vi "7HP_EnFlo_Specific - USB.vi"(5 "Datalog file path (full)":path, 6 "COM port":refnum<visa-resource-name>, 7 "Log data stream":bool, 8 "Set data rate (Hz)":u8(ring)=14 items=["1", "2", "4", "5", "8", "10", "16", "20", "25", "32", "40", "50", "64", "80", "100", "125", "160", "200", "250", "320", "400", "500", "625", "800", "1000"], 9 "N samples":u32=1000, 10 "Command":T2="s") -> (0 "Error":errorcluster, 2 "All samples out":sgl[][](array[numeric]), 3 "Rendezvous out":bool)   [LabVIEW 2020]
uses:
  ctls/7HP_Cmd (USB).ctl
  Globals/Meas_global.vi
panel:
  in  "Main":T1(tab)
  out "Serial number":u32 format="%0d"
  out "Pressure sensor EEPROM checksums ok":bool[](array[boolean])
  out "Pressure sensor temperatures in range":bool[](array[boolean])
  out "Pressure sensor values in range":bool[](array[boolean])
  out "Subsystems ok":bool[](array[boolean])
  out "n":u16
  out "Auto zero progBar":u16(slide) caption="Collecting samples, please maintain dP = 0" scale=0.0..1000.0
  out "P_raw_Azero":sgl[](array[numeric])
  in  "EEPROM array 2":u16[](array[numeric])
  in  "EEPROM array":sgl[](array[numeric])
  out "Chk ok":bool
  out "EEPROM Checksum":u16 format="%04x"
  out "received":bool
  out "Returned data rate (Hz)":u16
  out "sent":bool
  out "Pitch (deg)":sgl format="%.2f"
  out "Roll (deg)":sgl format="%.2f"
  out "frm err":u32
  out "chk err":u32
  in  "Stop Data":bool
  out "Relative humidity (%)":sgl
  out "Env. sensor die temperature (deg C)":sgl
  out "External thermistor temperature (deg C)":sgl
  out "Atmospheric pressure (mbar)":sgl
  out "Checksum ok":bool
  out "Gyration vector (deg / s)":sgl[](array[numeric])
  out "Acceleration vector (g)":sgl[](array[numeric])
  out "Pressures":sgl[][](graph)
  out "Stream enabled":bool
  # "Paul Nathan 10/2020"
  # "Output array order:\nP0.... (Pa)\n.\n.\nP6.... (Pa)\nP_atmos (mbar)....\nT_ext (deg C)....\nT_env (deg C)....\nRH (%)....\nax (g)....\nay (g)....\naz (g)....\nwx (deg / s)....\nwy (deg / s)....\nwz (deg / s)...."
  # "Pressure sensor 0 EEPROM checksum okay"
  # "Pressure sensor 1 EEPROM checksum okay"
  # "Pressure sensor 2 EEPROM checksum okay"
  # "Pressure sensor 3 EEPROM checksum okay"
  # "Pressure sensor 4 EEPROM checksum okay"
  # "Pressure sensor 5 EEPROM checksum okay"
  # "Pressure sensor 6 EEPROM checksum okay"
  # "Pressure sensor 0 temperature in range"
  # "Pressure sensor 1 temperature in range"
  # "Pressure sensor 2 temperature in range"
  # "Pressure sensor 3 temperature in range"
  # "Pressure sensor 4 temperature in range"
  # "Pressure sensor 5 temperature in range"
  # "Pressure sensor 6 temperature in range"
  # "Pressure sensor 0 value in range"
  # "Pressure sensor 1 value in range"
  # "Pressure sensor 2 value in range"
  # "Pressure sensor 3 value in range"
  # "Pressure sensor 4 value in range"
  # "Pressure sensor 5 value in range"
  # "Pressure sensor 6 value in range"
  # "Environmental sensor present"
  # "Inertial sensor present"
  # "Accelerometer self test pass"
  # "Gyroscope self test pass"
  # "External thermistor value in range"
  # "MCU EEPROM checksum ok"
  # "of 1000"
  # "P0 raw auto-zero"
  # "P1 raw auto-zero"
  # "P2 raw auto-zero"
  # "P3 raw auto-zero"
  # "P4 raw auto-zero"
  # "P5 raw auto-zero"
  # "P6 raw auto-zero"
  # "Power-up defaults"
  # "P0 raw auto-zero"
  # "Data rate (Hz)"
  # "P1 raw auto-zero"
  # "TTL streaming"
  # "P2 raw auto-zero"
  # "USB streaming"
  # "P3 raw auto-zero"
  # "TTL stream contains full data"
  # "P4 raw auto-zero"
  # "Accelerometer range mode"
  # "P5 raw auto-zero"
  # "Gyroscope range mode"
  # "P6 raw auto-zero"
  # "IMU rate mode"
  # "Atmospheric pressure offset (Pa)"
  # "External thermistor temperature offset (deg C)"
  # "Serial number"
  # "TTL baud rate (bps)"
  # "Accelerometer vector magnitude scale factor"
  # "Gyroscope x component offset (deg / s)"
  # "Gyroscope y component offset (deg / s)"
  # "Gyroscope z component offset (deg / s)"
  # "w_x"
  # "w_y"
  # "w_z"
  # "a_x"
  # "a_y"
  # "a_z"
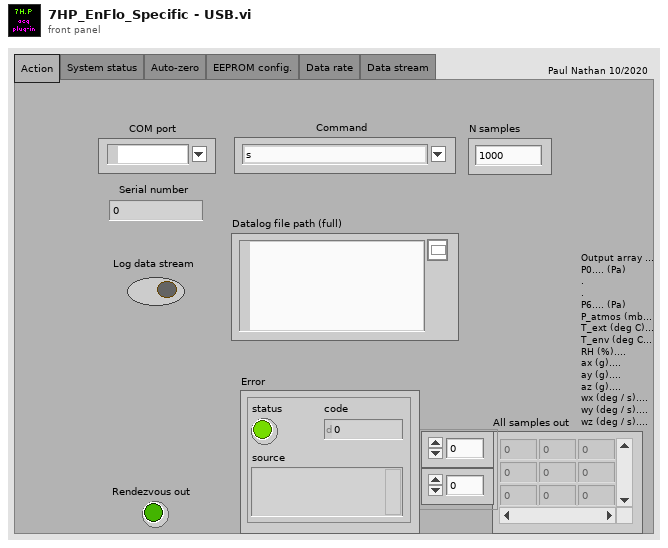
[diagram p1: front panel]
types:
  T1 = enum32{"Action", "System status", "Auto-zero", "EEPROM config.", "Data rate", "Data stream"}
  T2 = typedef "7HP_Cmd (USB).ctl" = string
  T3 = enum16{"open", "replace", "create", "open or create", "replace or create", "replace or create with confirmation"}
  T4 = typedef "Rendezvous RefNum" = refnum<k1>
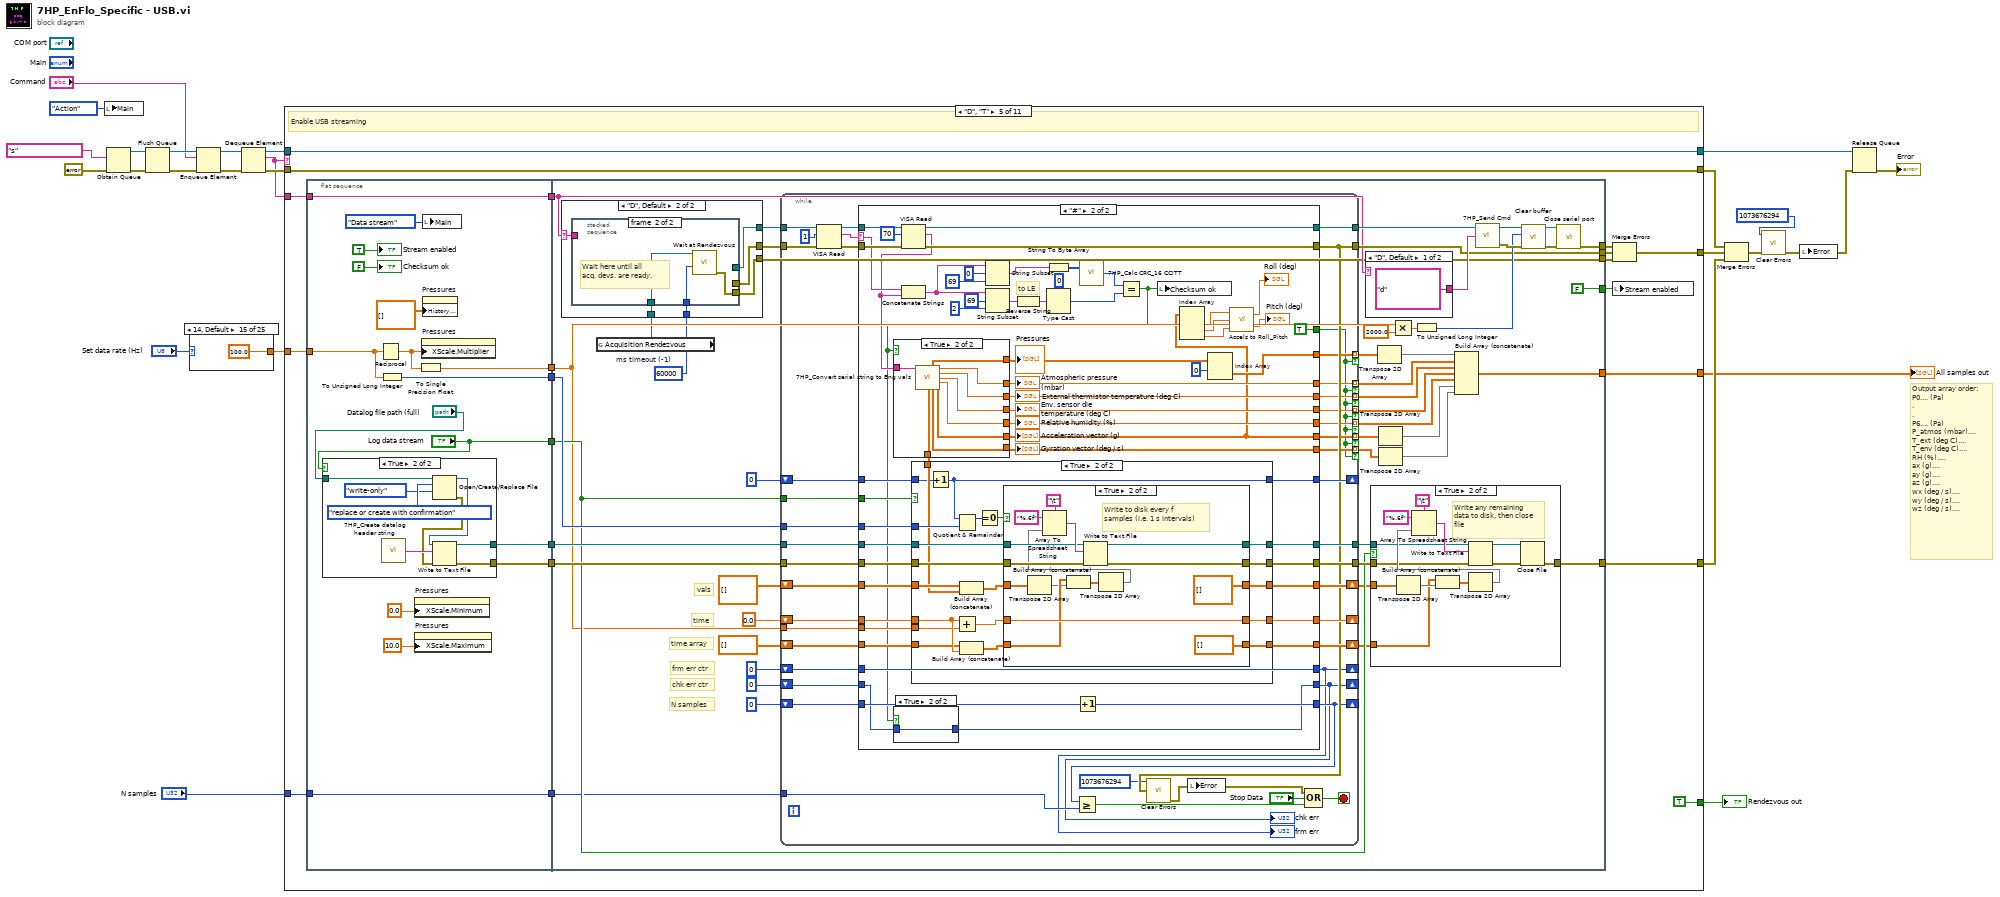
[diagram p0: block diagram]
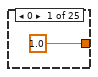
[diagram p2: hidden frame]
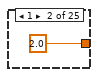
[diagram p3: hidden frame]
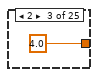
[diagram p4: hidden frame]
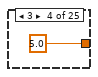
[diagram p5: hidden frame]
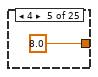
[diagram p6: hidden frame]
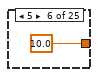
[diagram p7: hidden frame]
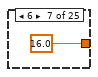
[diagram p8: hidden frame]
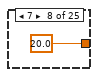
[diagram p9: hidden frame]
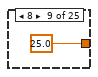
[diagram p10: hidden frame]
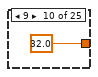
[diagram p11: hidden frame]
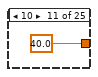
[diagram p12: hidden frame]
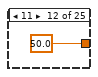
[diagram p13: hidden frame]
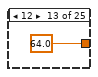
[diagram p14: hidden frame]
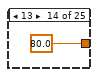
[diagram p15: hidden frame]
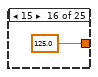
[diagram p16: hidden frame]
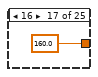
[diagram p17: hidden frame]
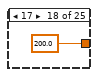
[diagram p18: hidden frame]
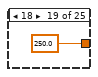
[diagram p19: hidden frame]
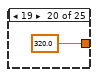
[diagram p20: hidden frame]
diagram:
  # "Output array order:\nP0.... (Pa)\n.\n.\nP6.... (Pa)\nP_atmos (mbar)....\nT_ext (deg C)....\nT_env (deg C)....\nRH (%)....\nax (g)....\nay (g)....\naz (g)....\nwx (deg / s)....\nwy (deg / s)....\nwz (deg / s)...."
  n1 = local write "Main"(T1."Action" ("Main")) -> ()
  n2 = Obtain Queue(element data type=T2 "s" ("Combo Box"), error in (no error)=errorcluster {"status"=FALSE, "code"=0, "source"=""}) -> (queue out=w24:refnum<queue>, error out=w25:errorcluster)  [unwired: 3 in, 1 out]
  n3 = Flush Queue(queue=w24, error in (no error)=w25) -> (queue out=w23:refnum<queue>, error out=w18:errorcluster)  [unwired: 1 out]
  n4 = case shown="14, Default" "Set data rate (Hz)" {
    tunnel: [1.0 2.0 4.0 5.0 8.0 10.0 16.0 20.0 25.0 32.0 40.0 50.0 64.0 80.0 100.0 125.0 160.0 200.0 250.0 320.0 400.0 500.0 625.0 800.0 1000.0] -> w3
    frame 0 {
    }
    frame 1 {
    }
    frame 2 {
    }
    frame 3 {
    }
    frame 4 {
    }
    frame 5 {
    }
    frame 6 {
    }
    frame 7 {
    }
    frame 8 {
    }
    frame 9 {
    }
    frame 10 {
    }
    frame 11 {
    }
    frame 12 {
    }
    frame 13 {
    }
    frame 14, Default {
    }
    frame 15 {
    }
    frame 16 {
    }
    frame 17 {
    }
    frame 18 {
    }
    frame 19 {
    }
    frame 20 {
    }
    frame 21 {
    }
    frame 22 {
    }
    frame 23 {
    }
    frame 24 {
    }
  }
  n5 = Enqueue Element(queue=w23, element="Command", error in (no error)=w18) -> (queue out=w19:refnum<queue>, error out=w17:errorcluster)  [unwired: 1 in, 1 out]
  n6 = Dequeue Element(queue=w19, error in (no error)=w17) -> (queue out=w14:refnum<queue>, element=w12:T2, error out=w13:errorcluster)  [unwired: 1 in, 1 out]
  n7 = case shown="\"D\", \"T\"" w12 {
    tunnel: w14 -> [w57 w96 w133 w210 w285 w592 w616 w670 w703 w726 w730]
    tunnel: [w57 w96 w133 w210 w285 w592 w616 w670 w703 w726 w730] -> w15
    tunnel: w13 -> [w56 w95 w132 w209 w284 w591 w617 w671 w702 w725 w729]
    tunnel: [w56 w95 w132 w209 w284 w591 w617 w671 w702 w725 w729] -> w11
    tunnel: w12 -> [w55 w94 w131 w208 w283 w594 w619 w673 w701 _ _]
    tunnel: [w53 w92 w129 w206 w268 w593 w618 w672 w699 errorcluster {"status"=FALSE, "code"=0, "source"=""} ("Error out") errorcluster {"status"=FALSE, "code"=0, "source"=""} ("Error out")] -> w10
    tunnel: [_ _ _ _ w281 _ _ _ _ _ _] -> w9
    tunnel: "N samples" -> [_ _ _ _ w274 _ _ _ _ _ _]
    tunnel: [_ _ _ _ w272 _ _ _ _ _ _] -> w5
    tunnel: w3 -> [_ _ _ _ w271 w589 _ _ _ _ _]
    tunnel: [FALSE FALSE FALSE FALSE TRUE FALSE FALSE FALSE FALSE FALSE FALSE] -> w1
    frame "S", "s" {
      # "Perform self-test and retrieve status bytes, Retrieve status bytes"
      n8 = flat-sequence {
        tunnel: w55 -> [w60]
        tunnel: [w60] -> w54
        tunnel: w54 -> [w66]
        tunnel: [w61] -> w53
        frame #0 {
          w59 = bool[] [] ("Pressure sensor EEPROM checksums ok")
          n9 = local write "Main"(T1."System status" ("Main")) -> ()
          "Pressure sensor EEPROM checksums ok" <- w59
          "Pressure sensor temperatures in range" <- w59
          "Pressure sensor values in range" <- w59
          "Subsystems ok" <- w59
        }
        frame #1 {
          w70 = 1 ("length (rest)")
          w78 = u8 0 ("byte count")
          n10 = local read "COM port"() -> (w67:refnum<visa-resource-name>)
          n11 = call "Open serial port.vi"("timeout (ms)"=u32 5000, "VISA resource name"=w67) -> ("Error out"=w88:errorcluster, "VISA resource name out"=w89:refnum<visa-resource-name>)  [unwired: 8 in]
          n12 = call "7HP_Send Cmd.vi"("Error In"=w88, "Operation"=w66, "Port"=w89) -> ("Error Out"=w86:errorcluster, "Port out"=w87:refnum<visa-resource-name>)  [unwired: 1 in]
          n13 = VISA Read(VISA resource name=w87, byte count=u32 4, error in (no error)=w86) -> (VISA resource name out=w84:refnum<visa-resource-name>, read buffer=w73:string, error out=w83:errorcluster)  [unwired: 1 out]
          n14 = call "Close serial port.vi"("Error in"=w83, "VISA resource name"=w84) -> ("Error out"=w61:errorcluster)  [unwired: 9 in]
          n15 = String Subset(string=w73, offset (0)=0, length (rest)=w70) -> (substring=w82:string)
          n16 = String Subset(string=w73, offset (0)=1, length (rest)=w70) -> (substring=w81:string)
          n17 = String Subset(string=w73, offset (0)=2 ("length (rest)"), length (rest)=w70) -> (substring=w80:string)
          n18 = String Subset(string=w73, offset (0)=3, length (rest)=w70) -> (substring=w79:string)
          n19 = Type Cast(type=w78, x=w82) -> (*(type *) &x=w77:u8)
          n20 = Type Cast(type=w78, x=w81) -> (*(type *) &x=w76:u8)
          n21 = Type Cast(type=w78, x=w80) -> (*(type *) &x=w75:u8)
          n22 = Type Cast(type=w78, x=w79) -> (*(type *) &x=w74:u8)
          n23 = Number To Boolean Array(number=w77) -> (Boolean array=w65:bool[])
          n24 = Number To Boolean Array(number=w76) -> (Boolean array=w64:bool[])
          n25 = Number To Boolean Array(number=w75) -> (Boolean array=w63:bool[])
          n26 = Number To Boolean Array(number=w74) -> (Boolean array=w62:bool[])
          n27 = local write "Pressure sensor EEPROM checksums ok"(w65) -> ()
          n28 = local write "Pressure sensor temperatures in range"(w64) -> ()
          n29 = local write "Pressure sensor values in range"(w63) -> ()
          n30 = local write "Subsystems ok"(w62) -> ()
        }
      }
    }
    frame "Z", "z" {
      # "Perform permanent auto-zero (write values to EEPROM), Perform temporary auto-zero"
      n31 = flat-sequence {
        tunnel: w94 -> [w100]
        tunnel: [w100] -> w93
        tunnel: w93 -> [w107]
        tunnel: [w103] -> w92
        frame #0 {
          n32 = local write "Main"(T1."Auto-zero" ("Main")) -> ()
          "P_raw_Azero" <- sgl[] [] ("P_raw_Azero")
          "Auto zero progBar" <- u16 0 ("Collecting samples, please maintain dP = 0")
        }
        frame #1 {
          n33 = local read "COM port"() -> (w108:refnum<visa-resource-name>)
          n34 = call "Open serial port.vi"("timeout (ms)"=u32 16000, "VISA resource name"=w108) -> ("Error out"=w114:errorcluster, "VISA resource name out"=w115:refnum<visa-resource-name>)  [unwired: 8 in]
          n35 = call "7HP_Send Cmd.vi"("Error In"=w114, "Operation"=w107, "Port"=w115) -> ("Error Out"=w112:errorcluster, "Port out"=w113:refnum<visa-resource-name>)  [unwired: 1 in]
          n36 = VISA Read(VISA resource name=w113, byte count=u32 28, error in (no error)=w112) -> (VISA resource name out=w110:refnum<visa-resource-name>, read buffer=w104:string, error out=w109:errorcluster)  [unwired: 1 out]
          n37 = for {
            N: 1000 -> [_]
            shift-right: [w117] -> _
            shift-left: u16 0 -> [w118]
            n38 = Increment(x=w118) -> (x+1=w117:u16)
            "n" <- w117
            n39 = Wait (ms)(milliseconds to wait=u32 11) -> ()  [unwired: 1 out]
            n40 = local write "Auto zero progBar"(w117) -> ()
          }
          n41 = for {
            N: 7 -> [_]
            tunnel: [w121] -> w106 mode=indexing
            tunnel: w104 -> [w120]
            i -> [w127]
            w125 = 4 ("x")
            # "to BE"
            n42 = Multiply(x=w125, y=w127) -> (x*y=w126:i32)
            n43 = String Subset(string=w120, offset (0)=w126, length (rest)=w125) -> (substring=w124:string)
            n44 = Reverse String(1:w124) -> (0:w123:string)
            n45 = Type Cast(type=sgl 0.0 ("byte count"), x=w123) -> (*(type *) &x=w121:sgl)
          }
          n46 = call "Close serial port.vi"("Error in"=w109, "VISA resource name"=w110) -> ("Error out"=w103:errorcluster)  [unwired: 9 in]
          n47 = local write "P_raw_Azero"(w106) -> ()
        }
      }
    }
    frame "R" {
      # "Read all EEPROM values"
      n48 = flat-sequence {
        tunnel: w131 -> [w137]
        tunnel: [w137] -> w130
        tunnel: w130 -> [w175]
        tunnel: [w174] -> w129
        frame #0 {
          n49 = local write "EEPROM array"(sgl[] [] ("EEPROM array")) -> ()
          n50 = local write "Main"(T1."EEPROM config." ("Main")) -> ()
          n51 = local write "EEPROM array 2"(u16[] [] ("EEPROM array 2")) -> ()
        }
        frame #1 {
          # "to BE"
          # "to BE"
          n52 = local read "COM port"() -> (w176:refnum<visa-resource-name>)
          n53 = call "Open serial port.vi"("timeout (ms)"=u32 5000, "VISA resource name"=w176) -> ("Error out"=w182:errorcluster, "VISA resource name out"=w183:refnum<visa-resource-name>)  [unwired: 8 in]
          n54 = call "7HP_Send Cmd.vi"("Error In"=w182, "Operation"=w175, "Port"=w183) -> ("Error Out"=w180:errorcluster, "Port out"=w181:refnum<visa-resource-name>)  [unwired: 1 in]
          n55 = VISA Read(VISA resource name=w181, byte count=u32 70, error in (no error)=w180) -> (VISA resource name out=w178:refnum<visa-resource-name>, read buffer=w142:string, error out=w177:errorcluster)  [unwired: 1 out]
          n56 = call "Close serial port.vi"("Error in"=w177, "VISA resource name"=w178) -> ("Error out"=w174:errorcluster)  [unwired: 9 in]
          n57 = String Subset(string=w142, offset (0)=0, length (rest)=48 ("length (rest)")) -> (substring=w145:string)
          n58 = String Subset(string=w142, offset (0)=56, length (rest)=12 ("length (rest)")) -> (substring=w150:string)
          n59 = String Subset(string=w142, offset (0)=48, length (rest)=2 ("length (rest)")) -> (substring=w159:string)
          n60 = String Subset(string=w142, offset (0)=50, length (rest)=6 ("length (rest)")) -> (substring=w163:string)
          n61 = String Subset(string=w142, offset (0)=68, length (rest)=2 ("length (rest)")) -> (substring=w170:string)
          n62 = String Subset(string=w142, offset (0)=0, length (rest)=68 ("length (rest)")) -> (substring=w173:string)
          n63 = for {
            N: 12 -> [_]
            tunnel: [w196] -> w151 mode=indexing
            tunnel: w145 -> [w195]
            i -> [w200]
            w198 = 4 ("x")
            # "to BE"
            n64 = Multiply(x=w198, y=w200) -> (x*y=w199:i32)
            n65 = String Subset(string=w195, offset (0)=w199, length (rest)=w198) -> (substring=w194:string)
            n66 = Reverse String(1:w194) -> (0:w193:string)
            n67 = Type Cast(type=sgl 0.0 ("byte count"), x=w193) -> (*(type *) &x=w196:sgl)
          }
          n68 = for {
            N: 3 -> [_]
            tunnel: [w188] -> w152 mode=indexing
            tunnel: w150 -> [w187]
            i -> [w192]
            w190 = 4 ("x")
            # "to BE"
            n69 = Multiply(x=w190, y=w192) -> (x*y=w191:i32)
            n70 = String Subset(string=w187, offset (0)=w191, length (rest)=w190) -> (substring=w186:string)
            n71 = Reverse String(1:w186) -> (0:w185:string)
            n72 = Type Cast(type=sgl 0.0 ("byte count"), x=w185) -> (*(type *) &x=w188:sgl)
          }
          n73 = Reverse String(1:w159) -> (0:w153:string)
          n74 = Reverse String(1:w170) -> (0:w166:string)
          n75 = String To Byte Array(string=w173) -> (unsigned byte array=w164:u8[])
          n76 = call "7HP_Calc CRC_16 CCITT.vi"("Data bytes"=w164) -> ("CRC_16-CCITT"=w165:u16)  [unwired: 1 in]
          n77 = Type Cast(type=u16 0 ("byte count"), x=w153) -> (*(type *) &x=w160:u16)
          n78 = Type Cast(type=u16 0 ("byte count"), x=w166) -> (*(type *) &x=w139:u16)
          n79 = String To Byte Array(string=w163) -> (unsigned byte array=w161:u8[])
          n80 = To Unsigned Word Integer(number=w161) -> (unsigned 16bit integer=w162:u16[])
          n81 = Equal?(x=w139, y=w165) -> (x = y?=w138:bool)
          n82 = Build Array (concatenate)(w151, w152) -> (w140:sgl[])
          n83 = Build Array (concatenate)(w160, w162) -> (w141:u16[])
          n84 = local write "EEPROM array"(w140) -> ()
          n85 = local write "EEPROM array 2"(w141) -> ()
          n86 = local write "EEPROM Checksum"(w139) -> ()
          n87 = local write "Chk ok"(w138) -> ()
        }
      }
    }
    frame "W" {
      # "Write all EEPROM values (including new checksum)"
      n88 = flat-sequence {
        tunnel: w208 -> [w223]
        tunnel: [w223] -> w207
        tunnel: [w216] -> w204
        tunnel: [w213] -> w203
        tunnel: [w212] -> w202
        tunnel: [w211] -> w201
        tunnel: w207 -> [w249]
        tunnel: [w248] -> w206
        tunnel: w204 -> [w229]
        tunnel: w203 -> [w226]
        tunnel: w202 -> [w228]
        tunnel: w201 -> [w227]
        frame #0 {
          n89 = local write "Main"(T1."EEPROM config." ("Main")) -> ()
          n90 = Split 1D Array(array="EEPROM array", index=12) -> (first subarray=w216:sgl[], second subarray=w213:sgl[])
          n91 = Split 1D Array(array="EEPROM array 2", index=1) -> (first subarray=w219:u16[], second subarray=w220:u16[])
          n92 = Index Array(array=w219, index=0) -> (element=w212:u16)
          n93 = To Unsigned Byte Integer(number=w220) -> (unsigned 8bit integer=w211:u8[])
        }
        frame #1 {
          # "to LE"
          # "to LE"
          n94 = local read "COM port"() -> (w250:refnum<visa-resource-name>)
          n95 = for {
            N: 12 -> [_]
            tunnel: w229 -> [w262] mode=indexing
            shift-right: [w263] -> w233
            shift-left: "" -> [w264]
            # "to LE"
            n96 = Type Cast(type="", x=w262) -> (*(type *) &x=w261:string)
            n97 = Reverse String(1:w261) -> (0:w260:string)
            n98 = Concatenate Strings(w264, w260) -> (w263:string)
          }
          n99 = for {
            N: 3 -> [_]
            tunnel: w226 -> [w256] mode=indexing
            shift-right: [w257] -> w240
            shift-left: "" -> [w258]
            # "to LE"
            n100 = Type Cast(type="", x=w256) -> (*(type *) &x=w255:string)
            n101 = Reverse String(1:w255) -> (0:w254:string)
            n102 = Concatenate Strings(w258, w254) -> (w257:string)
          }
          n103 = Type Cast(type="", x=w228) -> (*(type *) &x=w237:string)
          n104 = Reverse String(1:w237) -> (0:w239:string)
          n105 = call "Open serial port.vi"("timeout (ms)"=u32 5000, "VISA resource name"=w250) -> ("Error out"=w251:errorcluster, "VISA resource name out"=w252:refnum<visa-resource-name>)  [unwired: 8 in]
          n106 = Byte Array To String(unsigned byte array=w227) -> (string=w241:string)
          n107 = Concatenate Strings(w233, w239, w241, w240) -> (w234:string)
          n108 = String To Byte Array(string=w234) -> (unsigned byte array=w242:u8[])
          n109 = call "7HP_Calc CRC_16 CCITT.vi"("Data bytes"=w242) -> ("CRC_16-CCITT"=w224:u16)  [unwired: 1 in]
          "EEPROM Checksum" <- w224
          n110 = Type Cast(type="", x=w224) -> (*(type *) &x=w243:string)
          n111 = Reverse String(1:w243) -> (0:w244:string)
          n112 = Concatenate Strings(w234, w244) -> (w225:string)
          n113 = call "7HP_Send Cmd + Data.vi"("Error In"=w251, "Data"=w225, "Operation"=w249, "Port"=w252) -> ("Error Out"=w247:errorcluster, "Port out"=w246:refnum<visa-resource-name>)  [unwired: 1 in]
          n114 = call "Close serial port.vi"("Error in"=w247, "VISA resource name"=w246) -> ("Error out"=w248:errorcluster)  [unwired: 9 in]
          "Chk ok" <- TRUE ("Chk ok")
        }
      }
    }
    frame "D", "T" {
      # "Enable USB streaming"
      n115 = flat-sequence {
        tunnel: w283 -> [w301]
        tunnel: [w301] -> w282
        tunnel: [w298] -> w280
        tunnel: [w297] -> w279
        tunnel: [w295] -> w278
        tunnel: w271 -> [w296]
        tunnel: [w293] -> w277
        tunnel: ["Log data stream"] -> w276
        tunnel: w274 -> [w289]
        tunnel: [w289] -> w273
        tunnel: w282 -> [w319]
        tunnel: [w358] -> w269
        tunnel: [w357] -> w281
        tunnel: w280 -> [w354]
        tunnel: w279 -> [w353]
        tunnel: w278 -> [w355]
        tunnel: w277 -> [w321]
        tunnel: w276 -> [w347]
        tunnel: [FALSE] -> w275
        tunnel: w273 -> [w334]
        tunnel: [w323] -> w272
        tunnel: [w320] -> w270
        tunnel: [w316] -> w267
        frame #0 {
          n116 = case shown="True" "Log data stream" {
            tunnel: "Datalog file path (full)" -> [_ w311]
            tunnel: [refnum<file> refnum ("refnum out") w305] -> w298
            tunnel: [errorcluster {"status"=FALSE, "code"=0, "source"=""} ("error out") w304] -> w297
            frame False {
            }
            frame True {
              n117 = call "7HP_Create datalog header string.vi"() -> ("Datalog header string"=w307:string)  [unwired: 1 in]
              n118 = Open/Create/Replace File(file path (use dialog)=w311, operation (0:open)=T3."replace or create with confirmation", access (0:read/write)=enum16{"read/write", "read-only", "write-only"}."write-only") -> (refnum out=w308:refnum<file>, error out=w306:errorcluster)  [unwired: 3 in, 1 out]
              n119 = Write to Text File(file (use dialog)=w308, text=w307, error in=w306) -> (refnum out=w305:refnum<file>, error out=w304:errorcluster)  [unwired: 1 in, 1 out]
            }
          }
          n120 = Reciprocal(x=w296) -> (1/x=w294:dbl)
          n121 = To Unsigned Long Integer(number=w296) -> (unsigned 32bit integer=w295:u32)
          n122 = property on="Pressures" class="WFChart (strict)"("XScale.Minimum"=0.0 ("X Scale.Range:Minimum")) -> ()  [unwired: 2 in, 2 out]
          n123 = property on="Pressures" class="WFChart (strict)"("XScale.Maximum"=10.0 ("X Scale.Range:Maximum")) -> ()  [unwired: 2 in, 2 out]
          n124 = To Single Precision Float(number=w294) -> (single precision float=w293:sgl)
          n125 = property on="Pressures" class="WFChart (strict)"("XScale.Multiplier"=w294) -> ()  [unwired: 2 in, 2 out]
          n126 = local write "Main"(T1."Data stream" ("Main")) -> ()
          n127 = property on="Pressures" class="WFChart (strict)"("History Data"=sgl[][] []) -> ()  [unwired: 2 in, 2 out]
          "Checksum ok" <- FALSE ("Checksum ok")
          "Stream enabled" <- TRUE ("Stream enabled")
        }
        frame #1 {
          w314 = 60000  # ms timeout (-1)
          # "N samples"
          # "chk err ctr"
          # "frm err ctr"
          # "vals"
          # "time"
          # "time array"
          n128 = global read "Meas_global.vi" "Acquisition Rendezvous"() -> (w315:T4)
          n129 = case shown="\"D\", Default" w319 {
            selector: w319 -> [w364 w380]
            tunnel: [w363 w379] -> w317
            tunnel: [w362 w378] -> w318
            tunnel: [w361 w377] -> w316
            tunnel: w315 -> [w360 w376]
            tunnel: w314 -> [w359 w375]
            frame "T" {
              n130 = stacked-sequence {
                tunnel: w364 -> [w367 _]
                tunnel: [w366 _] -> w363
                tunnel: [w365 _] -> w362
                tunnel: [_ w374] -> w361
                tunnel: w360 -> [_ w373]
                tunnel: w359 -> [_ w372]
                frame #0 {
                  n131 = local read "COM port"() -> (w368:refnum<visa-resource-name>)
                  n132 = call "Open serial port.vi"("timeout (ms)"=u32 15000, "VISA resource name"=w368) -> ("Error out"=w371:errorcluster, "VISA resource name out"=w370:refnum<visa-resource-name>)  [unwired: 8 in]
                  n133 = call "7HP_Send Cmd, wait for ack.vi"("Error In"=w371, "Operation"=w367, "Port"=w370) -> ("Error Out"=w366:errorcluster, "Port out"=w365:refnum<visa-resource-name>)  [unwired: 1 out]
                }
                frame #1 {
                  # "Wait here until all acq. devs. are ready."
                  n134 = call <vilib>:"Wait at Rendezvous.vi"("ms timeout (-1)"=w372, "rendezvous"=w373) -> ("error out"=w374:errorcluster)  [unwired: 3 in, 2 out]
                }
              }
            }
            frame "D", Default {
              n135 = stacked-sequence {
                tunnel: w380 -> [w384 _]
                tunnel: [w381 _] -> w379
                tunnel: [w382 _] -> w378
                tunnel: [_ w390] -> w377
                tunnel: w376 -> [_ w389]
                tunnel: w375 -> [_ w388]
                frame #0 {
                  n136 = local read "COM port"() -> (w386:refnum<visa-resource-name>)
                  n137 = call "Open serial port.vi"("timeout (ms)"=u32 15000, "VISA resource name"=w386) -> ("Error out"=w383:errorcluster, "VISA resource name out"=w385:refnum<visa-resource-name>)  [unwired: 8 in]
                  n138 = call "7HP_Send Cmd.vi"("Error In"=w383, "Operation"=w384, "Port"=w385) -> ("Error Out"=w381:errorcluster, "Port out"=w382:refnum<visa-resource-name>)  [unwired: 1 in]
                }
                frame #1 {
                  # "Wait here until all acq. devs. are ready."
                  n139 = call <vilib>:"Wait at Rendezvous.vi"("ms timeout (-1)"=w388, "rendezvous"=w389) -> ("error out"=w390:errorcluster)  [unwired: 3 in, 2 out]
                }
              }
            }
          }
          n140 = while {
            tunnel: [w426] -> w320
            tunnel: w318 -> [w427]
            tunnel: [w445] -> w346
            shift-right: [w441] -> _
            shift-left: u32 0 -> [w442]
            tunnel: w355 -> [w440]
            tunnel: w354 -> [w439]
            tunnel: w353 -> [w438]
            tunnel: [w437] -> w352
            tunnel: [w436] -> w351
            shift-right: [w435] -> w337
            shift-left: sgl[][] [] -> [w434]
            shift-right: [w431] -> _
            shift-left: sgl 0.0 ("Numeric") -> [w433]
            tunnel: w321 -> [w432]
            shift-right: [w429] -> w336
            shift-left: sgl[] [] -> [w430]
            tunnel: w347 -> [w428]
            shift-right: [w420] -> _
            shift-left: u32 0 -> [w423]
            tunnel: w334 -> [w422]
            tunnel: [w419] -> w333 mode=indexing if=w412
            tunnel: [w418] -> w329 mode=indexing if=w412
            tunnel: [w417] -> w328 mode=indexing if=w412
            tunnel: [w416] -> w327 mode=indexing if=w412
            tunnel: [w415] -> w326 mode=indexing if=w412
            tunnel: [w414] -> w331 mode=indexing if=w412
            tunnel: [w413] -> w330 mode=indexing if=w412
            tunnel: w317 -> [w411]
            shift-right: [w407] -> _
            shift-left: u32 0 -> [w409]
            shift-right: [w408] -> _
            shift-left: u32 0 -> [w410]
            stop <- w443 stop-if-true
            n141 = VISA Read(VISA resource name=w427, byte count=u32 1, error in (no error)=w411) -> (VISA resource name out=w447:refnum<visa-resource-name>, read buffer=w448:string, error out=w446:errorcluster)  [unwired: 1 out]
            n142 = case shown="\"#\"" w448 {
              selector: w448 -> [_ w513]
              tunnel: w447 -> [w461 w517]
              tunnel: [w462 w515] -> w426
              tunnel: w446 -> [w462 w518]
              tunnel: [w461 w516] -> w445
              tunnel: w442 -> [w460 w487]
              tunnel: [w460 w473] -> w441
              tunnel: w440 -> [_ w485]
              tunnel: w439 -> [w459 w484]
              tunnel: w438 -> [w458 w483]
              tunnel: [w458 w475] -> w437
              tunnel: [w459 w474] -> w436
              tunnel: [w457 w476] -> w435
              tunnel: w434 -> [w457 w482]
              tunnel: w433 -> [w456 w481]
              tunnel: w432 -> [_ w480]
              tunnel: [w456 w477] -> w431
              tunnel: w430 -> [w455 w479]
              tunnel: [w455 w478] -> w429
              tunnel: w428 -> [_ w486]
              tunnel: w423 -> [w454 w512]
              tunnel: [w454 w511] -> w420
              tunnel: [_ w510] -> w419
              tunnel: [FALSE TRUE] -> w412
              tunnel: [_ w509] -> w418
              tunnel: [_ w508] -> w417
              tunnel: [_ w507] -> w416
              tunnel: [_ w506] -> w415
              tunnel: [_ w468] -> w414
              tunnel: [_ w505] -> w413
              tunnel: w410 -> [w450 w470]
              tunnel: w409 -> [w452 w472]
              tunnel: [w451 w472] -> w407
              tunnel: [w450 w469] -> w408
              frame Default {
                n143 = Increment(x=w452) -> (x+1=w451:u32)
              }
              frame "#" {
                # "to LE"
                n144 = VISA Read(VISA resource name=w517, byte count=u32 70, error in (no error)=w518) -> (VISA resource name out=w516:refnum<visa-resource-name>, read buffer=w502:string, error out=w515:errorcluster)  [unwired: 1 out]
                n145 = Concatenate Strings(w513, w502) -> (w491:string)
                n146 = String Subset(string=w491, offset (0)=0, length (rest)=69 ("length (rest)")) -> (substring=w497:string)
                n147 = String Subset(string=w491, offset (0)=69, length (rest)=2 ("length (rest)")) -> (substring=w500:string)
                n148 = Reverse String(1:w500) -> (0:w499:string)
                n149 = String To Byte Array(string=w497) -> (unsigned byte array=w490:u8[])
                n150 = Type Cast(type=u16 0 ("length (rest)"), x=w499) -> (*(type *) &x=w498:u16)
                n151 = Increment(x=w512) -> (x+1=w511:u32)
                n152 = call "7HP_Calc CRC_16 CCITT.vi"("Data bytes"=w490) -> ("CRC_16-CCITT"=w489:u16)  [unwired: 1 in]
                n153 = Equal?(x=w489, y=w498) -> (x = y?=w471:bool)
                n154 = case shown="True" w471 {
                  tunnel: [w578 w587] -> w509
                  tunnel: [w578 w586] -> w508
                  tunnel: [w578 w585] -> w507
                  tunnel: [w578 w584] -> w506
                  tunnel: [w571 w583] -> w468
                  tunnel: [w571 w582] -> w505
                  tunnel: [w569 w581] -> w488
                  tunnel: [w577 w580] -> w504
                  tunnel: w502 -> [_ w579]
                  frame False {
                    w578 = sgl nan ("Atmospheric pressure (mbar)")
                    n155 = Initialize Array(sgl nan ("element"), 7 ("dimension size")) -> (w576:sgl[])
                    n156 = Initialize Array(sgl nan ("element"), 3 ("dimension size")) -> (w571:sgl[])
                    n157 = Initialize Array(sgl nan ("element"), 17 ("dimension size")) -> (w569:sgl[])
                    n158 = Build Array(w576) -> (w577:sgl[][])
                  }
                  frame True {
                    n159 = call "7HP_Convert serial string to Eng vals.vi"("Serial buffer string (excluding FrameChar)"=w579) -> ("Pressures"=w580:sgl[][], "Atmospheric pressure (mbar)"=w587:sgl, "External thermistor temperature (deg C)"=w586:sgl, "Env. sensor die temperature (deg C)"=w585:sgl, "Relative humidity (%)"=w584:sgl, "All vals"=w581:sgl[], "Gyration vector (deg / s)"=w582:sgl[], "Acceleration vector (g)"=w583:sgl[])  [unwired: 7 in]
                  }
                }
                "Pressures" <- w504
                "Acceleration vector (g)" <- w468
                "Gyration vector (deg / s)" <- w505
                "Atmospheric pressure (mbar)" <- w509
                "External thermistor temperature (deg C)" <- w508
                "Env. sensor die temperature (deg C)" <- w507
                "Relative humidity (%)" <- w506
                n160 = case shown="True" w471 {
                  tunnel: w470 -> [w520 w521]
                  tunnel: [w519 w521] -> w469
                  frame False {
                    n161 = Increment(x=w520) -> (x+1=w519:u32)
                  }
                  frame True {
                  }
                }
                n162 = case shown="True" w486 {
                  tunnel: w487 -> [w527 w529]
                  tunnel: [w527 w528] -> w473
                  tunnel: w485 -> [_ w547]
                  tunnel: w488 -> [_ w533]
                  tunnel: w484 -> [w525 w544]
                  tunnel: w483 -> [w526 w543]
                  tunnel: [w526 w542] -> w475
                  tunnel: [w525 w541] -> w474
                  tunnel: w482 -> [w524 w534]
                  tunnel: [w524 w540] -> w476
                  tunnel: w481 -> [w523 w537]
                  tunnel: w480 -> [_ w536]
                  tunnel: [w523 w539] -> w477
                  tunnel: w479 -> [w522 w535]
                  tunnel: [w522 w538] -> w478
                  frame False {
                  }
                  frame True {
                    n163 = Increment(x=w529) -> (x+1=w528:u32)
                    n164 = Add(x=w537, y=w536) -> (x+y=w532:sgl)
                    n165 = Quotient & Remainder(x=w528, y=w547) -> (x-y*floor(x/y)=w546:u32)  [unwired: 1 out]
                    n166 = Build Array (concatenate)(w534, w533) -> (w530:sgl[][])
                    n167 = Build Array (concatenate)(w535, w537) -> (w531:sgl[])
                    n168 = Equal To 0?(x=w546) -> (x = 0?=w545:bool)
                    n169 = case shown="True" w545 {
                      tunnel: w544 -> [w551 w564]
                      tunnel: w543 -> [w552 w563]
                      tunnel: [w552 w562] -> w542
                      tunnel: [w551 w561] -> w541
                      tunnel: w530 -> [w549 w556]
                      tunnel: [w549 sgl[][] []] -> w540
                      tunnel: w532 -> [w550 w559]
                      tunnel: [w550 w559] -> w539
                      tunnel: w531 -> [w548 w558]
                      tunnel: [w548 sgl[] []] -> w538
                      frame False {
                      }
                      frame True {
                        # "Write to disk every f samples (i.e. 1 s intervals)"
                        n170 = Transpose 2D Array(2D array=w556) -> (transposed array=w555:sgl[][])
                        n171 = Build Array (concatenate)(w558, w555) -> (w554:sgl[][])
                        n172 = Transpose 2D Array(2D array=w554) -> (transposed array=w553:sgl[][])
                        n173 = Array To Spreadsheet String(delimiter (Tab)="\t", array=w553, 3:"%.6f" ("format string")) -> (spreadsheet string=w567:string)
                        n174 = Write to Text File(file (use dialog)=w564, text=w567, error in=w563) -> (refnum out=w561:refnum<file>, error out=w562:errorcluster)  [unwired: 1 in, 1 out]
                      }
                    }
                  }
                }
                n175 = local write "Checksum ok"(w471) -> ()
                n176 = Index Array(array=w468) -> (element #1=w467:sgl, element #2=w466:sgl, element #3=w465:sgl)  [unwired: 3 in]
                n177 = Index Array(array=w504, index (row)=0) -> (element=w510:sgl[])  [unwired: 1 in]
                n178 = call "Accels to Roll_Pitch.vi"("az"=w465, "ay"=w466, "ax"=w467) -> ("Pitch (deg)"=→"Pitch (deg)":sgl, "Roll (deg)"=→"Roll (deg)":sgl)
              }
            }
            "chk err" <- w408
            "frm err" <- w407
            n179 = Greater Or Equal?(x=w420, y=w422) -> (x >= y?=w421:bool)
            n180 = call <vilib>:"Clear Errors.vi"("error in (no error)"=w426, "specific error code to clear (0: all)"=1073676294) -> ("error out"=w425:errorcluster)  [unwired: 4 in, 1 out]
            n181 = local write "Error"(w425) -> ()
            n182 = Compound Arithmetic op=OR(w425, "Stop Data", w421) -> (w443:bool)
          }
          n183 = case shown="\"D\", Default" w319 {
            tunnel: [T2 "d" ("Combo Box") T2 "t" ("Combo Box")] -> w322
            frame "D", Default {
            }
            frame "T" {
            }
          }
          n184 = case shown="True" w347 {
            tunnel: [w393 w406] -> w357
            tunnel: w352 -> [w393 w398]
            tunnel: w351 -> [_ w399]
            tunnel: w337 -> [_ w397]
            tunnel: w336 -> [_ w396]
            frame False {
            }
            frame True {
              # "Write any remaining data to disk, then close file"
              n185 = Transpose 2D Array(2D array=w397) -> (transposed array=w403:sgl[][])
              n186 = Build Array (concatenate)(w396, w403) -> (w404:sgl[][])
              n187 = Transpose 2D Array(2D array=w404) -> (transposed array=w405:sgl[][])
              n188 = Array To Spreadsheet String(delimiter (Tab)="\t", array=w405, 3:"%.6f" ("format string")) -> (spreadsheet string=w400:string)
              n189 = Write to Text File(file (use dialog)=w399, text=w400, error in=w398) -> (refnum out=w395:refnum<file>, error out=w394:errorcluster)  [unwired: 1 in, 1 out]
              n190 = Close File(refnum=w395, error in=w394) -> (error out=w406:errorcluster)  [unwired: 1 out]
            }
          }
          n191 = Transpose 2D Array(2D array=w333) -> (transposed array=w332:sgl[][])
          n192 = Transpose 2D Array(2D array=w331) -> (transposed array=w325:sgl[][])
          n193 = Transpose 2D Array(2D array=w330) -> (transposed array=w324:sgl[][])
          n194 = Multiply(x=w321, y=sgl 2000.0) -> (x*y=w340:sgl)
          n195 = To Unsigned Long Integer(number=w340) -> (unsigned 32bit integer=w338:u32)
          n196 = Build Array (concatenate)(w332, w329, w328, w327, w326, w325, w324) -> (w323:sgl[][])
          n197 = call "7HP_Send Cmd.vi"("Operation"=w322, "Port"=w346) -> ("Error Out"=w343:errorcluster, "Port out"=w344:refnum<visa-resource-name>)  [unwired: 2 in]
          n198 = call "Clear buffer.vi"("Error in"=w343, "dt for timeout (ms)"=w338, "VISA resource name in"=w344) -> ("Error out"=w341:errorcluster, "VISA resource name out"=w342:refnum<visa-resource-name>)  [unwired: 3 in]
          n199 = call "Close serial port.vi"("Error in"=w341, "VISA resource name"=w342) -> ("Error out"=w358:errorcluster)  [unwired: 9 in]
        }
      }
      n200 = Merge Errors(w269, w270, w267) -> (w268:errorcluster)
      n201 = local write "Stream enabled"(w275) -> ()
    }
    frame "d", "t" {
      # "Disable USB streaming"
      n202 = flat-sequence {
        tunnel: [w602] -> w595
        tunnel: w594 -> [w602]
        tunnel: w589 -> [w597]
        tunnel: [w596] -> w590
        tunnel: w595 -> [w610]
        tunnel: [w609] -> w593
        tunnel: w590 -> [w604]
        frame #0 {
          n203 = disable-structure shown="Disabled" {
            frame Disabled {
              n204 = local write "Main"(T1."Data stream" ("Main")) -> ()
            }
            frame Enabled {
            }
          }
          n205 = Reciprocal(x=w597) -> (1/x=w601:dbl)
          n206 = To Single Precision Float(number=w601) -> (single precision float=w599:sgl)
          n207 = Multiply(x=w599, y=sgl 2000.0) -> (x*y=w600:sgl)
          n208 = To Unsigned Long Integer(number=w600) -> (unsigned 32bit integer=w596:u32)
        }
        frame #1 {
          n209 = local read "COM port"() -> (w611:refnum<visa-resource-name>)
          n210 = call "Open serial port.vi"("timeout (ms)"=u32 5000, "VISA resource name"=w611) -> ("Error out"=w612:errorcluster, "VISA resource name out"=w613:refnum<visa-resource-name>)  [unwired: 8 in]
          n211 = call "7HP_Send Cmd.vi"("Error In"=w612, "Operation"=w610, "Port"=w613) -> ("Error Out"=w606:errorcluster, "Port out"=w608:refnum<visa-resource-name>)  [unwired: 1 in]
          n212 = call "Clear buffer.vi"("Error in"=w606, "dt for timeout (ms)"=w604, "VISA resource name in"=w608) -> ("Error out"=w605:errorcluster, "VISA resource name out"=w607:refnum<visa-resource-name>)  [unwired: 3 in]
          n213 = call "Close serial port.vi"("Error in"=w605, "VISA resource name"=w607) -> ("Error out"=w609:errorcluster)  [unwired: 9 in]
        }
      }
    }
    frame "F" {
      # "Set data rate"
      n214 = flat-sequence {
        tunnel: [w626] -> w620
        tunnel: w619 -> [w626]
        tunnel: [w633] -> w621
        tunnel: w620 -> [w631]
        tunnel: w621 -> [w667]
        tunnel: [w667] -> w618
        frame #0 {
          n215 = local write "Returned data rate (Hz)"(u16 0 ("Returned data rate (Hz)")) -> ()
          n216 = local write "received"(FALSE ("received")) -> ()
          n217 = local write "Main"(T1."Data rate" ("Main")) -> ()
          n218 = local write "sent"(FALSE ("sent")) -> ()
        }
        frame #1 {
          # "to LE"
          n219 = local read "Set data rate (Hz)"() -> (w629:u8)
          n220 = case shown="14, Default" w629 {
            tunnel: [1.0 2.0 4.0 5.0 8.0 10.0 16.0 20.0 25.0 32.0 40.0 50.0 64.0 80.0 100.0 125.0 160.0 200.0 250.0 320.0 400.0 500.0 625.0 800.0 1000.0] -> w628
            frame 0 {
            }
            frame 1 {
            }
            frame 2 {
            }
            frame 3 {
            }
            frame 4 {
            }
            frame 5 {
            }
            frame 6 {
            }
            frame 7 {
            }
            frame 8 {
            }
            frame 9 {
            }
            frame 10 {
            }
            frame 11 {
            }
            frame 12 {
            }
            frame 13 {
            }
            frame 14, Default {
            }
            frame 15 {
            }
            frame 16 {
            }
            frame 17 {
            }
            frame 18 {
            }
            frame 19 {
            }
            frame 20 {
            }
            frame 21 {
            }
            frame 22 {
            }
            frame 23 {
            }
            frame 24 {
            }
          }
          n221 = local read "COM port"() -> (w632:refnum<visa-resource-name>)
          n222 = To Unsigned Word Integer(number=w628) -> (unsigned 16bit integer=w635:u16)
          n223 = call "Open serial port.vi"("timeout (ms)"=u32 5000, "VISA resource name"=w632) -> ("Error out"=w638:errorcluster, "VISA resource name out"=w637:refnum<visa-resource-name>)  [unwired: 8 in]
          n224 = Type Cast(type="", x=w635) -> (*(type *) &x=w634:string)
          n225 = Reverse String(1:w634) -> (0:w630:string)
          n226 = call "7HP_Send Cmd + Data.vi"("Error In"=w638, "Data"=w630, "Operation"=w631, "Port"=w637) -> ("Error Out"=w640:errorcluster, "Port out"=w639:refnum<visa-resource-name>)  [unwired: 1 in]
          n227 = call "Close serial port.vi"("Error in"=w640, "VISA resource name"=w639) -> ("Error out"=w633:errorcluster)  [unwired: 9 in]
        }
        frame #2 {
          n228 = Unbundle By Name(w667) -> ("status"=w668:bool)
          n229 = Not(x=w668) -> (.not. x?=→"sent":bool)
        }
      }
    }
    frame "f" {
      # "Get data rate"
      n230 = flat-sequence {
        tunnel: [w679] -> w674
        tunnel: w673 -> [w679]
        tunnel: [w691] -> w675
        tunnel: w674 -> [w689]
        tunnel: w675 -> [w696]
        tunnel: [w696] -> w672
        frame #0 {
          n231 = local write "received"(FALSE ("received")) -> ()
          n232 = local write "Main"(T1."Data rate" ("Main")) -> ()
          n233 = local write "sent"(FALSE ("sent")) -> ()
        }
        frame #1 {
          # "to BE"
          n234 = local read "COM port"() -> (w690:refnum<visa-resource-name>)
          n235 = call "Open serial port.vi"("timeout (ms)"=u32 5000, "VISA resource name"=w690) -> ("Error out"=w694:errorcluster, "VISA resource name out"=w693:refnum<visa-resource-name>)  [unwired: 8 in]
          n236 = call "7HP_Send Cmd.vi"("Error In"=w694, "Operation"=w689, "Port"=w693) -> ("Error Out"=w683:errorcluster, "Port out"=w684:refnum<visa-resource-name>)  [unwired: 1 in]
          n237 = VISA Read(VISA resource name=w684, byte count=u32 2, error in (no error)=w683) -> (VISA resource name out=w681:refnum<visa-resource-name>, read buffer=w687:string, error out=w682:errorcluster)  [unwired: 1 out]
          n238 = Reverse String(1:w687) -> (0:w685:string)
          n239 = call "Close serial port.vi"("Error in"=w682, "VISA resource name"=w681) -> ("Error out"=w691:errorcluster)  [unwired: 9 in]
          n240 = Type Cast(type=u16 0 ("byte count"), x=w685) -> (*(type *) &x=→"Returned data rate (Hz)":u16)
        }
        frame #2 {
          n241 = Unbundle By Name(w696) -> ("status"=w697:bool)
          n242 = Not(x=w697) -> (.not. x?=→"received":bool)
        }
      }
    }
    frame "N" {
      # "Get serial number"
      n243 = flat-sequence {
        tunnel: w701 -> [w706]
        tunnel: [w706] -> w700
        tunnel: w700 -> [w713]
        tunnel: [w712] -> w699
        frame #0 {
          n244 = local write "Main"(T1."Action" ("Main")) -> ()
          "Serial number" <- u32 0 ("Numeric")
        }
        frame #1 {
          # "to BE"
          n245 = local read "COM port"() -> (w714:refnum<visa-resource-name>)
          n246 = call "Open serial port.vi"("timeout (ms)"=u32 5000, "VISA resource name"=w714) -> ("Error out"=w720:errorcluster, "VISA resource name out"=w721:refnum<visa-resource-name>)  [unwired: 8 in]
          n247 = call "7HP_Send Cmd.vi"("Error In"=w720, "Operation"=w713, "Port"=w721) -> ("Error Out"=w718:errorcluster, "Port out"=w719:refnum<visa-resource-name>)  [unwired: 1 in]
          n248 = VISA Read(VISA resource name=w719, byte count=u32 4, error in (no error)=w718) -> (VISA resource name out=w716:refnum<visa-resource-name>, read buffer=w709:string, error out=w715:errorcluster)  [unwired: 1 out]
          n249 = call "Close serial port.vi"("Error in"=w715, "VISA resource name"=w716) -> ("Error out"=w712:errorcluster)  [unwired: 9 in]
          n250 = Reverse String(1:w709) -> (0:w710:string)
          n251 = Type Cast(type=sgl 0.0 ("byte count"), x=w710) -> (*(type *) &x=w708:sgl)
          n252 = To Unsigned Long Integer(number=w708) -> (unsigned 32bit integer=w707:u32)
          n253 = local write "Serial number"(w707) -> ()
        }
      }
    }
    frame "X" {
      # "Exit"
    }
    frame Default {
    }
  }
  "All samples out" <- w5
  "Rendezvous out" <- w1
  n254 = Merge Errors(w11, w10, w9) -> (w8:errorcluster)
  n255 = call <vilib>:"Clear Errors.vi"("error in (no error)"=w8, "specific error code to clear (0: all)"=1073676294) -> ("error out"=w16:errorcluster)  [unwired: 4 in, 1 out]
  n256 = local write "Error"(w16) -> ()
  n257 = Release Queue(queue=w15, error in (no error)=w16) -> (error out=→"Error":errorcluster)  [unwired: 1 in, 2 out]
